vi "AES-KeyExpansion.vi"(8 "error in (no error)":errorcluster, 11 "Key In":u8[](array[numeric]) format="%.0x") -> (0 "error out":errorcluster, 3 "Expanded Key [U8]":u8[](array[numeric]) format="%02x")   [LabVIEW 2011, in "i3-external-encryption.lvlib"]
doc: "Expands a Key using AES Key expansion.\n\n(c) Ton Plomp, 2011\nTHIS SOFTWARE IS PROVIDED AS IS, AND ANY WARRANTY IS REJECTED"
uses:
  i3-external-encryption.lvlib
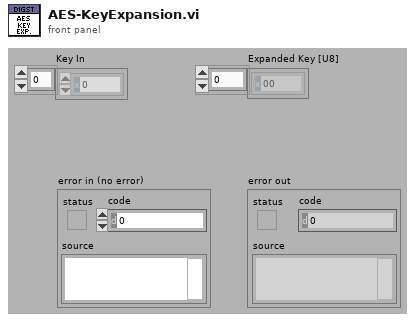
[diagram p1: front panel]
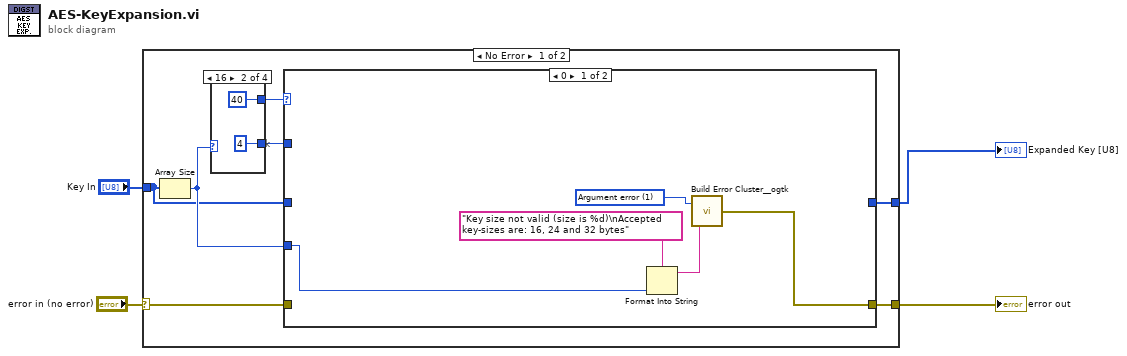
[diagram p0: block diagram]
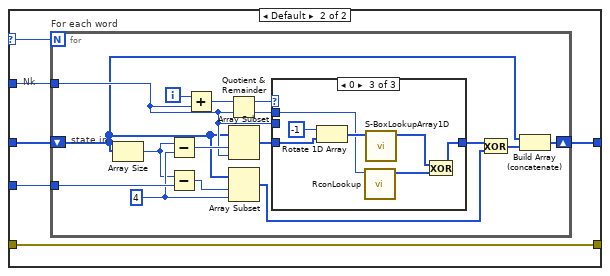
[diagram p2: hidden frame]
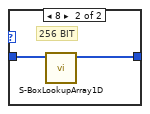
[diagram p5: hidden frame]
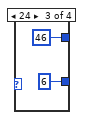
[diagram p7: hidden frame]
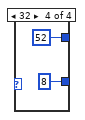
[diagram p8: hidden frame]
diagram:
  n1 = case shown="No Error" "error in (no error)" {
    selector: "error in (no error)" -> [w6 w59]
    tunnel: [w9 _] -> w4
    tunnel: "Key In" -> [w5 _]
    tunnel: [w7 w59] -> w2
    frame No Error {
      # "Nk"
      n2 = Array Size(array=w5) -> (size(s)=w11:i32)
      n3 = case shown="16" w11 {
        tunnel: [_ 40 46 52] -> w8
        tunnel: [_ 4 6 8] -> w10
        frame 0, Default {
        }
        frame 16 {
        }
        frame 24 {
        }
        frame 32 {
        }
      }
      n4 = case shown="0" w8 {
        selector: w8 -> [_ w17]
        tunnel: w11 -> [w12 w22]
        tunnel: w10 -> [_ w21]
        tunnel: [_ w20] -> w9
        tunnel: w5 -> [_ w19]
        tunnel: w6 -> [_ w18]
        tunnel: [w15 w18] -> w7
        frame 0 {
          w16 = 1 items=["No error", "Argument error", "Memory is full", "Out of zone", "End of file", "File already open", "Generic file I/O error", "File not found", "File permission error", "Disk is full", "Duplicate path", "Too many files open", "System feature not enabled", "Resource file not found", "Cannot add resource", "Resource not found", "Image not found", "Image memory error", "Pen does not exist", "Config type invalid", "Config token not found", "Config parse error", "Config memory error", "Bad external code format", "Bad external code offset", "External code not present", "Null window", "Destroy window error", "Null menu", "Print aborted", "Bad print record", "Print driver error", "Windows error during printing", "Memory error during printing", "Print dialog error", "Generic print error", "Invalid device refnum", "Device not found", "Device parameter error", "Device unit error", "Cannot open device", "Device call aborted", "Generic error", "Cancelled by user", "Object ID too low", "Object ID too high", "Object not in heap", "Unknown heap", "Unknown object (invalid DefProc)", "Unknown object (DefProc not in table)", "Message out of range", "Invalid (null) method", "Unknown message", "Manager call not supported", "Bad address", "Network operation in progress", "Network operation timed out", "Connection is busy", "Network attribute not supported", "Network error", "Address in use", "System out of memory", "Connection aborted", "Connection refused", "Not connected", "Already connected", "Connection closed", "Initialization error (interapplication manager)", "Bad occurrence", "Wait on unbound occurrence handler", "Occurrence queue overflow", "Datalog type conflict", "Unused", "Unrecognized type (interapplication manager)", "Memory corrupt", "Failed to make temporary DLL", "Old CIN version", "Drag socket not found", "Failed to load drop-object", "Failed to register OLE object", "Failed to release OLE object", "Format specifier type mismatch", "Unknown format specifier", "Too few format specifiers", "Too many format specifiers", "Scan failed", "Newer CIN version", "Error converting to variant", "Runtime menu error", "Password tampered", "Variant attribute not found", "Incompatible variant data type", "Event data is not available", "Event Store is not present", "Occurrence is not found", "Event Queue is not created", "Event info is not available", "Refnum passed is NULL", "Error retrieving Class GUID", "Error retrieving CoClass GUID", "Error retrieving TypeLib GUID.", "Bad built application magic bytes.", "Specific driver is different from the specific driver associated with the Logical Name.", "There is no session opened to the class driver.", "Max Error", "MAX - Error with config objects", "MAX - Error loading configuration", "MAX - Group not supported"]
          n5 = Format Into String(format string="Key size not valid (size is %d)\nAccepted key-sizes are: 16, 24 and 32 bytes" ("String to Prepend to source (\"\")"), w12) -> (resulting string=w13:string)  [unwired: 2 in, 1 out]
          n6 = call <userlib>:"Build Error Cluster__ogtk.vi"("String to Prepend to source (\"\")"=w13, "code"=w16) -> ("error out"=w15:errorcluster)
        }
        frame Default {
          # "Nk"
          n7 = for "For each word" {
            N: w17 -> [_]
            shift-right: [w38] -> w20
            shift-left: w19 -> [w25]
            tunnel: w22 -> [w37]
            tunnel: w21 -> [w26]
            i -> [w34]
            w29 = 4 ("y")
            # "state in"
            n8 = Array Size(array=w25) -> (size(s)=w23:i32)
            n9 = Subtract(x=w23, y=w29) -> (x-y=w36:i32)
            n10 = Subtract(x=w23, y=w37) -> (x-y=w24:i32)
            n11 = Add(x=w34, y=w26) -> (x+y=w30:i32)
            n12 = Quotient & Remainder(x=w30, y=w26) -> (x-y*floor(x/y)=w35:i32, floor(x/y)=w27:i32)
            n13 = Array Subset(array=w25, index=w36, length=w26) -> (w31:u8[])
            n14 = Array Subset(array=w25, index=w24, length=w29) -> (w33:u8[])
            n15 = case shown="0" w35 {
              tunnel: w31 -> [w39 w40 w51]
              tunnel: [w39 w41 w46] -> w32
              tunnel: w26 -> [_ w42 _]
              tunnel: w27 -> [_ _ w47]
              frame Default {
              }
              frame 4 {
                n16 = case shown="Default" w42 {
                  tunnel: [w43 w44] -> w41
                  tunnel: w40 -> [w43 w45]
                  frame Default {
                  }
                  frame 8 {
                    # "256 BIT"
                    n17 = call "S-BoxLookupArray1D.vi"("In"=w45) -> ("Out"=w44:u8[])  [unwired: 10 in]
                  }
                }
              }
              frame 0 {
                n18 = Rotate 1D Array(1:w51, 2:-1 ("n")) -> (0:w49:u8[])
                n19 = call "RconLookup.vi"("iteration"=w47) -> ("LookUp-Out"=w50:u8[])  [unwired: 10 in]
                n20 = call "S-BoxLookupArray1D.vi"("In"=w49) -> ("Out"=w48:u8[])  [unwired: 10 in]
                n21 = Exclusive Or(1:w50, 2:w48) -> (0:w46:u8[])
              }
            }
            n22 = Exclusive Or(1:w33, 2:w32) -> (0:w28:u8[])
            n23 = Build Array (concatenate)(w25, w28) -> (w38:u8[])
          }
        }
      }
    }
    frame Error {
    }
  }
  "Expanded Key [U8]" <- w4
  "error out" <- w2
